vi "Chad Magic Voodoo 2.vi"() -> ()   [LabVIEW 2016]
panel:
  in  "Automatic Wire\n Feed not to Exceed":dbl=1.4
  in  "Add Wire Feed... (%)":dbl=4.0
  in  "For Every... (mm)":dbl=0.2
  out "W trigger Y":dbl
  out "C trigger Y":dbl
  out "R trigger Y":dbl
  in  "Window Bead Trigger heights":dbl[](array[numeric])
  in  "Robot Bead Trigger heights":dbl[](array[numeric])
  in  "Center Bead Trigger heights":dbl[](array[numeric])
  out "Shutter Open":bool
  in  "base path":path=path "C:/Users/Mark/Desktop/BeadScan"
  in  "Write Code":bool
  out "Bead3 Size":i32
  out "Bead2 Size":i32
  out "Bead1 Size":i32
  in  "Tab Control":T1(tab)
  in  "Mark Target Bead Height":bool
  out "All Beads":cluster{dbl[], dbl[]}[](graph)
  out "Target Bead Height":dbl
  in  "Set Correction C":bool
  in  "Set Trigger Offset":dbl
  in  "Center Bead Corrections":dbl[](array[numeric])
  in  "Center Bead Trigger Positions":dbl[](array[numeric])
  out "Center Bead #1":cluster{dbl[], dbl[]}[](graph)
  out "Center Bead Trigger":dbl
  in  "Set Trigger Center":bool
  in  "Undo":bool
  out "Difference From Bead Height Setpoint C":dbl
  out "Recommended % Change\n in Wire Feed C":dbl
  in  "Set Correction R":bool
  in  "Set Trigger Offset 2":dbl
  out "Robot Bead #2":cluster{dbl[], dbl[]}[](graph)
  in  "Robot Bead Trigger Positions":dbl[](array[numeric])
  in  "Robot Bead Corrections":dbl[](array[numeric])
  out "Robot Bead Trigger":dbl
  in  "Set Trigger Robot":bool
  in  "Undo":bool
  out "Difference From Bead Height Setpoint R":dbl
  out "Recommended % Change\n in Wire Feed R":dbl
  in  "Set Correction W":bool
  in  "Set Trigger Offset 3":dbl
  out "Window Bead #3":cluster{dbl[], dbl[]}[](graph)
  in  "Window Bead Trigger Positions":dbl[](array[numeric])
  in  "Window Bead Corrections":dbl[](array[numeric])
  out "Window Bead Trigger":dbl
  in  "Set Trigger Window":bool
  in  "Undo":bool
  out "Difference From Bead Height Setpoint W":dbl
  out "Recommended % Change\n in Wire Feed W":dbl
  in  "stop":bool
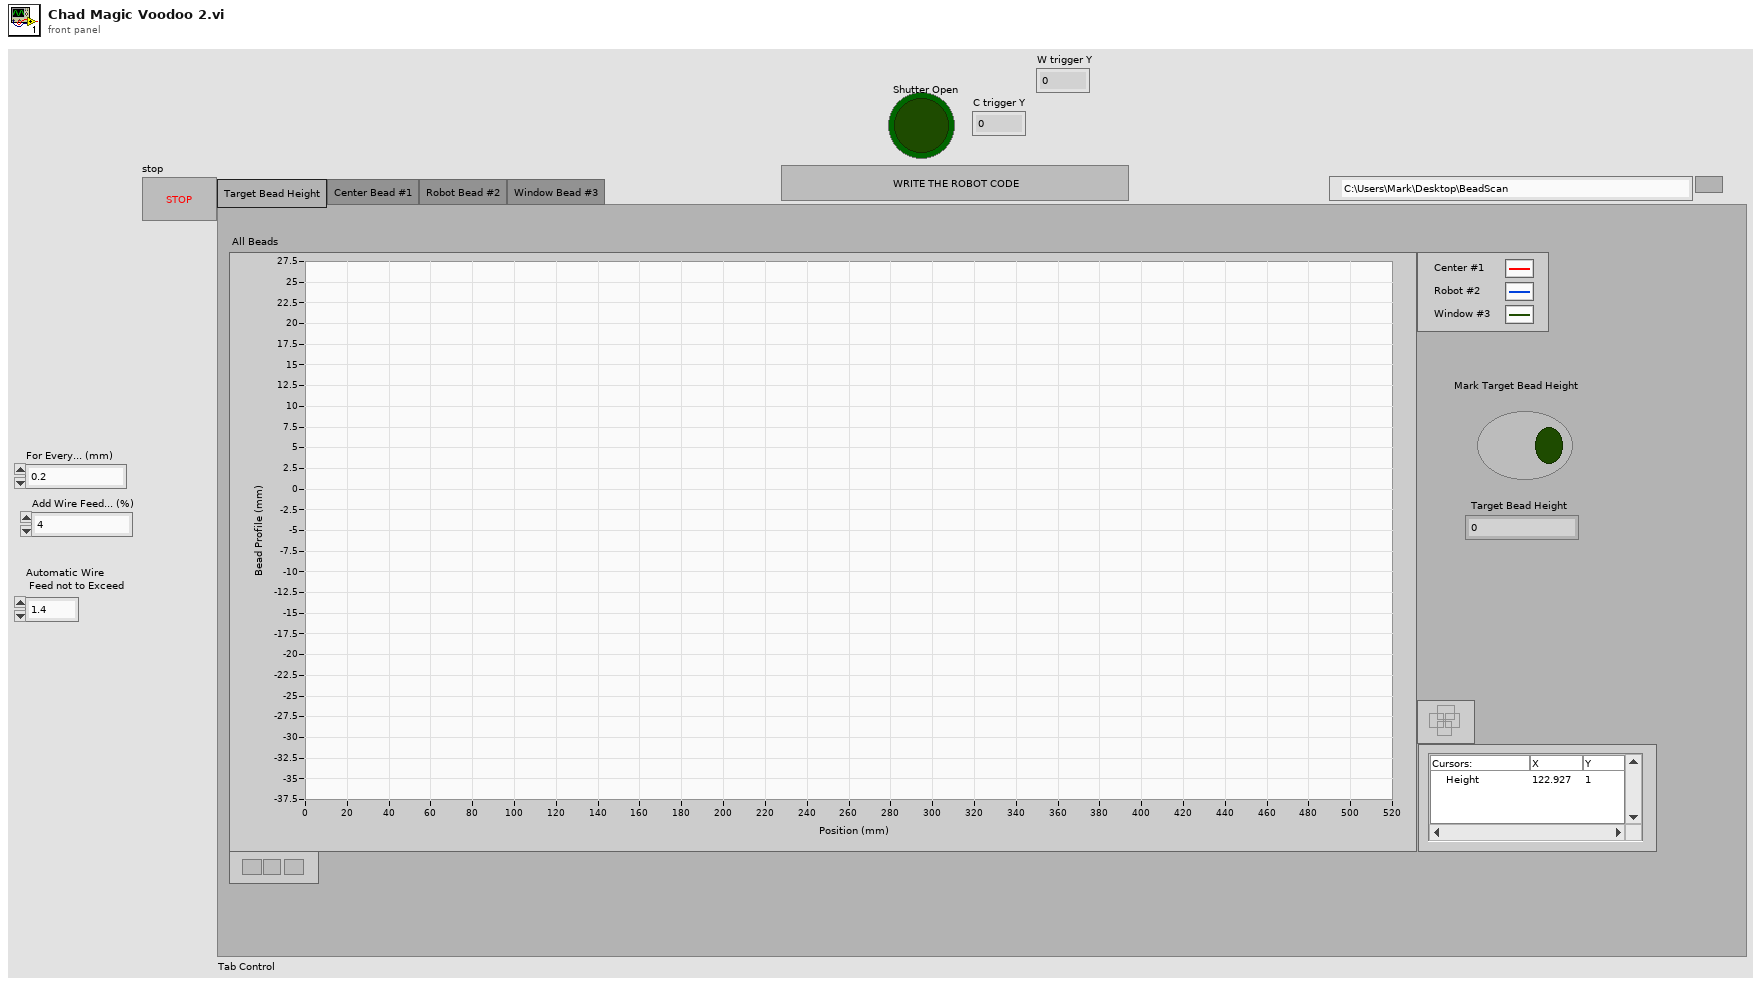
[diagram p1: front panel]
types:
  T1 = enum32{"Target Bead Height", "Center Bead #1", "Robot Bead #2", "Window Bead #3"}
  T2 = enum16{"open", "replace", "create", "open or create", "replace or create", "replace or create with confirmation"}
  T3 = cluster{"[0]":cluster{dbl[], dbl[]}, "[1]":cluster{dbl[], dbl[]}, "[2]":cluster{dbl[], dbl[]}}
  T4 = cluster{dbl[], "Center Bead Trigger heights":dbl[]}
  T5 = cluster{dbl[], "Window Bead Trigger heights":dbl[]}
  T6 = cluster{dbl[], "Robot Bead Trigger heights":dbl[]}
  T7 = cluster{dbl[], "Center Bead Trigger heights":dbl[]}[]
  T8 = cluster{dbl[], "Robot Bead Trigger heights":dbl[]}[]
  T9 = cluster{dbl[], "Window Bead Trigger heights":dbl[]}[]
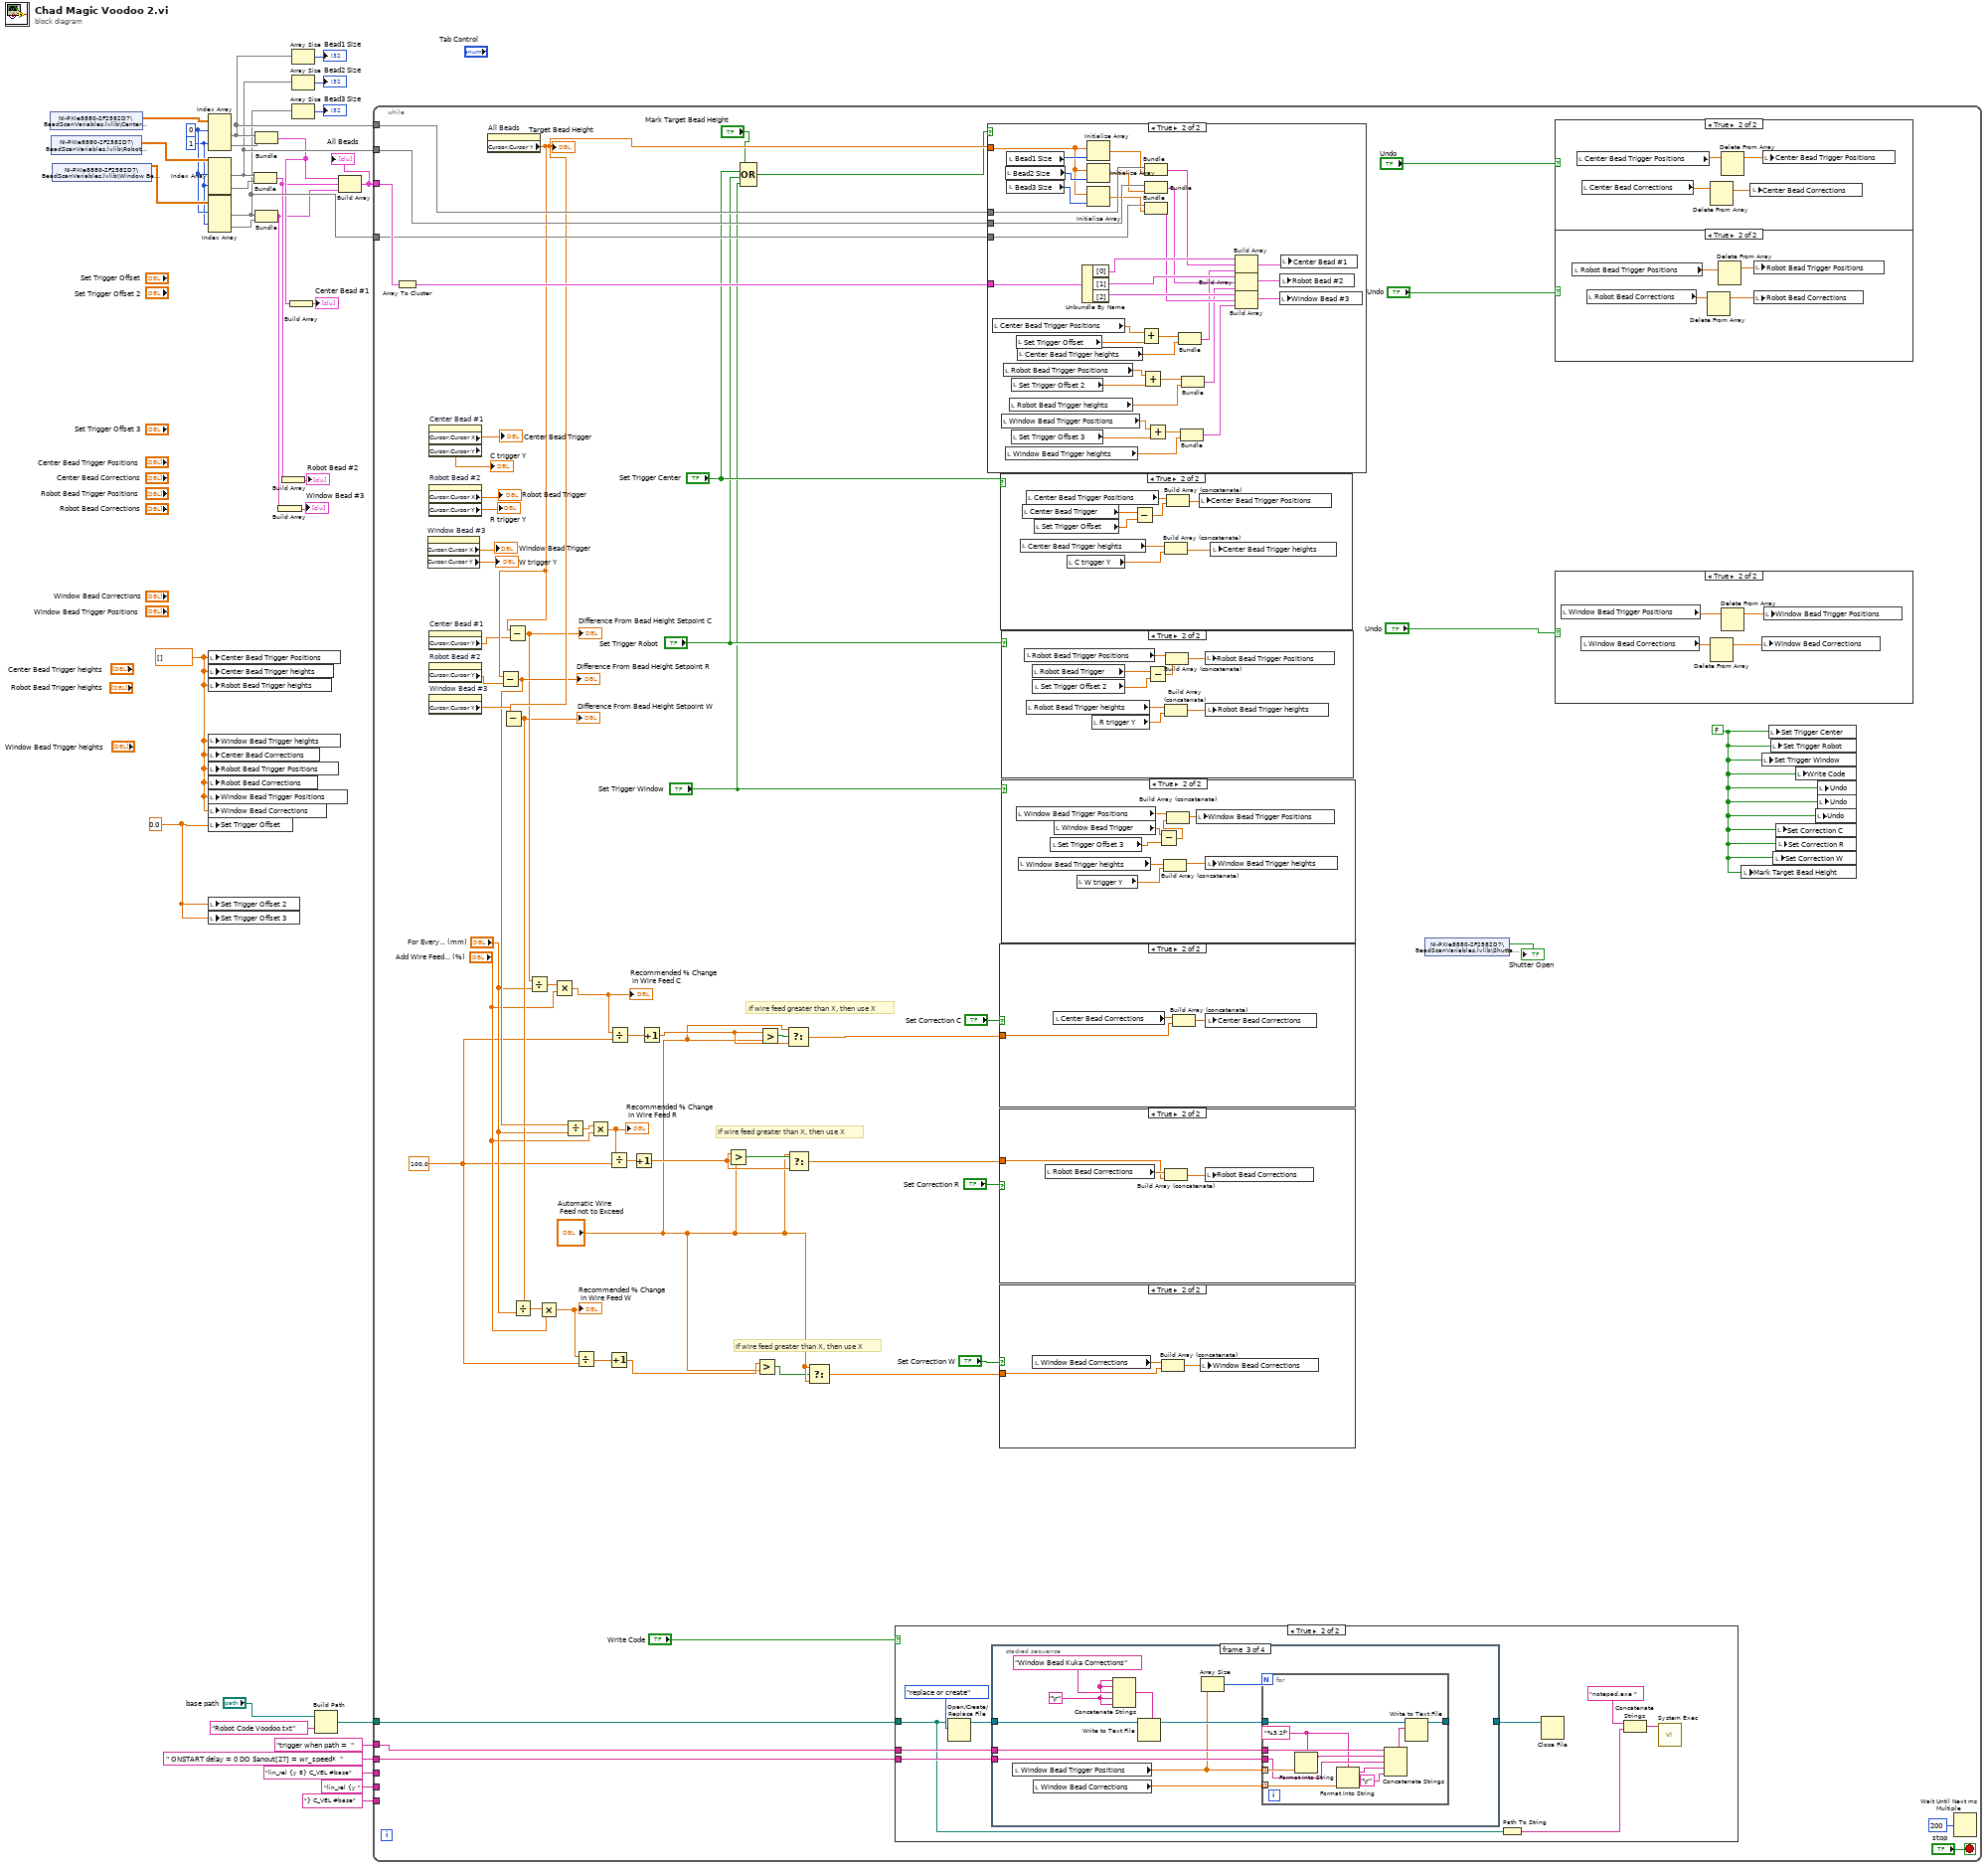
[diagram p0: block diagram]
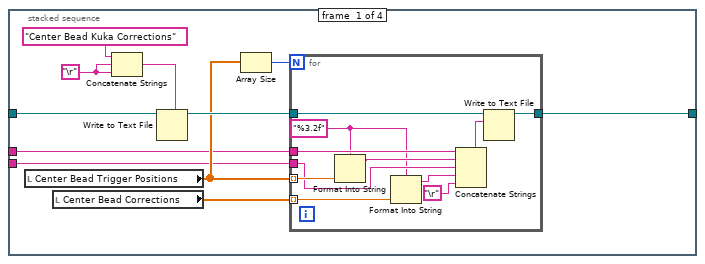
[diagram p6: hidden frame]
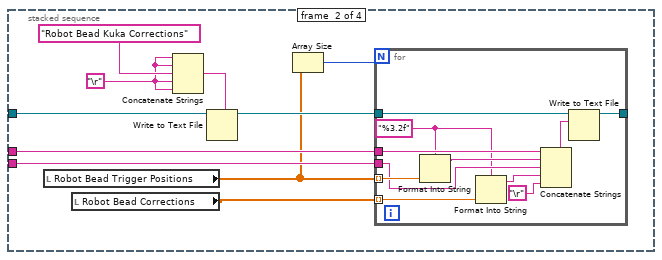
[diagram p7: hidden frame]
diagram:
  w2 = 0.0
  w1 = dbl[] []
  w26 = 1 ("index (row)")
  w27 = 0 ("index (row)")
  n1 = shared-variable "NI-PXIe8880-2F2582D7\\BeadScanVariables.lvlib\\Center Bead #1"() -> (w31:dbl[][])  [unwired: 1 in, 1 out]
  n2 = shared-variable "NI-PXIe8880-2F2582D7\\BeadScanVariables.lvlib\\Robot Bead #2"() -> (w29:dbl[][])  [unwired: 1 in, 1 out]
  n3 = shared-variable "NI-PXIe8880-2F2582D7\\BeadScanVariables.lvlib\\Window Bead #3"() -> (w28:dbl[][])  [unwired: 1 in, 1 out]
  n4 = Index Array(array=w31, index (row) #1=w27, index (row) #2=w26) -> (element #1=w19:dbl[], element #2=w30:dbl[])  [unwired: 2 in]
  n5 = Index Array(array=w29, index (row) #1=w27, index (row) #2=w26) -> (element #1=w18:dbl[], element #2=w25:dbl[])  [unwired: 2 in]
  n6 = Index Array(array=w28, index (row) #1=w27, index (row) #2=w26) -> (element #1=w17:dbl[], element #2=w24:dbl[])  [unwired: 2 in]
  n7 = local write "Center Bead Trigger Positions"(w1) -> ()
  n8 = local write "Center Bead Trigger heights"(w1) -> ()
  n9 = local write "Robot Bead Trigger heights"(w1) -> ()
  n10 = local write "Window Bead Trigger heights"(w1) -> ()
  n11 = local write "Center Bead Corrections"(w1) -> ()
  n12 = local write "Robot Bead Trigger Positions"(w1) -> ()
  n13 = local write "Robot Bead Corrections"(w1) -> ()
  n14 = local write "Window Bead Trigger Positions"(w1) -> ()
  n15 = local write "Window Bead Corrections"(w1) -> ()
  n16 = local write "Set Trigger Offset"(w2) -> ()
  n17 = local write "Set Trigger Offset 2"(w2) -> ()
  n18 = local write "Set Trigger Offset 3"(w2) -> ()
  n19 = Bundle(w18, w25) -> (w14:cluster{dbl[], dbl[]})  [unwired: 1 in]
  n20 = Bundle(w19, w30) -> (w15:cluster{dbl[], dbl[]})  [unwired: 1 in]
  n21 = Bundle(w17, w24) -> (w11:cluster{dbl[], dbl[]})  [unwired: 1 in]
  n22 = Build Array(w11) -> (→"Window Bead #3":cluster{dbl[], dbl[]}[])
  n23 = Build Array(w14) -> (→"Robot Bead #2":cluster{dbl[], dbl[]}[])
  n24 = Build Array(w15) -> (→"Center Bead #1":cluster{dbl[], dbl[]}[])
  n25 = Array Size(array=w19) -> (size(s)=→"Bead1 Size":i32)
  n26 = Array Size(array=w18) -> (size(s)=→"Bead2 Size":i32)
  n27 = Array Size(array=w17) -> (size(s)=→"Bead3 Size":i32)
  n28 = Build Path(base path="base path", name or relative path="Robot Code Voodoo.txt") -> (appended path=w8:path)
  n29 = Build Array(w15, w14, w11) -> (w20:cluster{dbl[], dbl[]}[])
  "All Beads" <- w20
  n30 = while {
    tunnel: w20 -> [w87]
    tunnel: w19 -> [w85]
    tunnel: w18 -> [w84]
    tunnel: w17 -> [w83]
    tunnel: w8 -> [w78]
    tunnel: "trigger when path =  " -> [w77]
    tunnel: " ONSTART delay = 0 DO $anout[27] = wr_speed*  " -> [w76]
    tunnel: "lin_rel {y 8} C_VEL #base" -> [_]
    tunnel: "lin_rel {y " -> [_]
    tunnel: "} C_VEL #base" -> [_]
    stop <- "stop" stop-if-true
    w46 = 100.0 ("y")
    w42 = FALSE
    # "If wire feed greater than X, then use X"
    # "If wire feed greater than X, then use X"
    # "If wire feed greater than X, then use X"
    n31 = Array To Cluster(array=w87) -> (cluster=w86:T3)
    n32 = property on="Window Bead #3" class="XYGraph (strict)"() -> ("Cursor.Cursor X"=→"Window Bead Trigger":dbl, "Cursor.Cursor Y"=→"W trigger Y":dbl)  [unwired: 2 in, 2 out]
    n33 = property on="Center Bead #1" class="XYGraph (strict)"() -> ("Cursor.Cursor X"=→"Center Bead Trigger":dbl, "Cursor.Cursor Y"=→"C trigger Y":dbl)  [unwired: 2 in, 2 out]
    n34 = property on="Robot Bead #2" class="XYGraph (strict)"() -> ("Cursor.Cursor X"=→"Robot Bead Trigger":dbl, "Cursor.Cursor Y"=→"R trigger Y":dbl)  [unwired: 2 in, 2 out]
    n35 = property on="Center Bead #1" class="XYGraph (strict)"() -> ("Cursor.Cursor Y"=w72:dbl)  [unwired: 2 in, 2 out]
    n36 = property on="Robot Bead #2" class="XYGraph (strict)"() -> ("Cursor.Cursor Y"=w71:dbl)  [unwired: 2 in, 2 out]
    n37 = property on="Window Bead #3" class="XYGraph (strict)"() -> ("Cursor.Cursor Y"=w70:dbl)  [unwired: 2 in, 2 out]
    n38 = property on="All Beads" class="XYGraph (strict)"() -> ("Cursor.Cursor Y"=w73:dbl)  [unwired: 2 in, 2 out]
    "Target Bead Height" <- w73
    n39 = Subtract(x=w73, y=w71) -> (x-y=w58:dbl)
    "Difference From Bead Height Setpoint R" <- w58
    n40 = Subtract(x=w73, y=w70) -> (x-y=w55:dbl)
    "Difference From Bead Height Setpoint W" <- w55
    n41 = Subtract(x=w73, y=w72) -> (x-y=w56:dbl)
    "Difference From Bead Height Setpoint C" <- w56
    n42 = Divide(x=w55, y="For Every... (mm)") -> (x/y=w59:dbl)
    n43 = Divide(x=w56, y="For Every... (mm)") -> (x/y=w57:dbl)
    n44 = Multiply(x=w59, y="Add Wire Feed... (%)") -> (x*y=w47:dbl)
    "Recommended % Change\n in Wire Feed W" <- w47
    n45 = Multiply(x=w57, y="Add Wire Feed... (%)") -> (x*y=w48:dbl)
    "Recommended % Change\n in Wire Feed C" <- w48
    n46 = Divide(x=w58, y="For Every... (mm)") -> (x/y=w60:dbl)
    n47 = Divide(x=w47, y=w46) -> (x/y=w43:dbl)
    n48 = Multiply(x=w60, y="Add Wire Feed... (%)") -> (x*y=w49:dbl)
    "Recommended % Change\n in Wire Feed R" <- w49
    n49 = Divide(x=w49, y=w46) -> (x/y=w45:dbl)
    n50 = Increment(x=w43) -> (x+1=w41:dbl)
    n51 = Divide(x=w48, y=w46) -> (x/y=w44:dbl)
    n52 = Increment(x=w45) -> (x+1=w36:dbl)
    n53 = Increment(x=w44) -> (x+1=w40:dbl)
    n54 = Greater?(x=w36, y="Automatic Wire\n Feed not to Exceed") -> (0:w37:bool)
    n55 = Compound Arithmetic op=OR("Mark Target Bead Height", "Set Trigger Center", "Set Trigger Robot", "Set Trigger Window") -> (w64:bool)
    n56 = Greater?(x=w41, y="Automatic Wire\n Feed not to Exceed") -> (0:w33:bool)
    n57 = Greater?(x=w40, y="Automatic Wire\n Feed not to Exceed") -> (0:w39:bool)
    n58 = Select(t="Automatic Wire\n Feed not to Exceed", s=w39, f=w40) -> (s? t:f=w38:dbl)
    n59 = Select(t="Automatic Wire\n Feed not to Exceed", s=w37, f=w36) -> (s? t:f=w35:dbl)
    n60 = Select(t="Automatic Wire\n Feed not to Exceed", s=w33, f="Automatic Wire\n Feed not to Exceed") -> (s? t:f=w32:dbl)
    n61 = case shown="True" "Write Code" {
      tunnel: w78 -> [_ w100]
      tunnel: w77 -> [_ w107]
      tunnel: w76 -> [_ w106]
      frame False {
      }
      frame True {
        n62 = Open/Create/Replace File(file path (use dialog)=w100, operation (0:open)=T2."replace or create") -> (refnum out=w108:refnum<file>)  [unwired: 4 in, 2 out]
        n63 = stacked-sequence {
          tunnel: w108 -> [w116 w137 w158 _]
          tunnel: w107 -> [w111 w135 w156 _]
          tunnel: w106 -> [w110 w134 w155 _]
          tunnel: [w109 _ _ _] -> w105
          frame #0 {
            w118 = "\r"
            n64 = local read "Center Bead Trigger Positions"() -> (w113:dbl[])
            n65 = local read "Center Bead Corrections"() -> (w112:dbl[])
            n66 = Concatenate Strings("Center Bead Kuka Corrections", w118, w118) -> (w117:string)
            n67 = Write to Text File(file (use dialog)=w116, text=w117) -> (refnum out=w115:refnum<file>)  [unwired: 2 in, 2 out]
            n68 = Array Size(array=w113) -> (size(s)=w114:i32)
            n69 = for {
              N: w114 -> [_]
              tunnel: w115 -> [w130]
              tunnel: w113 -> [w127] mode=indexing
              tunnel: w112 -> [w124] mode=indexing
              tunnel: w111 -> [w129]
              tunnel: w110 -> [w125]
              tunnel: [w122] -> w109
              w121 = "%3.2f" ("format string")
              n70 = Format Into String(format string=w121, w127) -> (resulting string=w128:string)  [unwired: 2 in, 1 out]
              n71 = Format Into String(format string=w121, w124) -> (resulting string=w123:string)  [unwired: 2 in, 1 out]
              n72 = Concatenate Strings(w129, w128, w125, w123, "\r") -> (w126:string)
              n73 = Write to Text File(file (use dialog)=w130, text=w126) -> (refnum out=w122:refnum<file>)  [unwired: 2 in, 2 out]
            }
          }
          frame #1 {
            w131 = "\r"
            n74 = local read "Robot Bead Trigger Positions"() -> (w132:dbl[])
            n75 = local read "Robot Bead Corrections"() -> (w133:dbl[])
            n76 = Concatenate Strings(w131, w131, "Robot Bead Kuka Corrections", w131, w131) -> (w139:string)
            n77 = Write to Text File(file (use dialog)=w137, text=w139) -> (refnum out=w138:refnum<file>)  [unwired: 2 in, 2 out]
            n78 = Array Size(array=w132) -> (size(s)=w136:i32)
            n79 = for {
              N: w136 -> [_]
              tunnel: w138 -> [w151]
              tunnel: w132 -> [w148] mode=indexing
              tunnel: w133 -> [w145] mode=indexing
              tunnel: w135 -> [w150]
              tunnel: w134 -> [w146]
              tunnel: [w143] -> _
              w142 = "%3.2f" ("format string")
              n80 = Format Into String(format string=w142, w148) -> (resulting string=w149:string)  [unwired: 2 in, 1 out]
              n81 = Format Into String(format string=w142, w145) -> (resulting string=w144:string)  [unwired: 2 in, 1 out]
              n82 = Concatenate Strings(w150, w149, w146, w144, "\r") -> (w147:string)
              n83 = Write to Text File(file (use dialog)=w151, text=w147) -> (refnum out=w143:refnum<file>)  [unwired: 2 in, 2 out]
            }
          }
          frame #2 {
            w152 = "\r"
            n84 = local read "Window Bead Trigger Positions"() -> (w153:dbl[])
            n85 = local read "Window Bead Corrections"() -> (w154:dbl[])
            n86 = Concatenate Strings(w152, w152, "Window Bead Kuka Corrections", w152, w152) -> (w160:string)
            n87 = Write to Text File(file (use dialog)=w158, text=w160) -> (refnum out=w159:refnum<file>)  [unwired: 2 in, 2 out]
            n88 = Array Size(array=w153) -> (size(s)=w157:i32)
            n89 = for {
              N: w157 -> [_]
              tunnel: w159 -> [w172]
              tunnel: w153 -> [w169] mode=indexing
              tunnel: w154 -> [w166] mode=indexing
              tunnel: w156 -> [w171]
              tunnel: w155 -> [w167]
              tunnel: [w164] -> _
              w163 = "%3.2f" ("format string")
              n90 = Format Into String(format string=w163, w169) -> (resulting string=w170:string)  [unwired: 2 in, 1 out]
              n91 = Format Into String(format string=w163, w166) -> (resulting string=w165:string)  [unwired: 2 in, 1 out]
              n92 = Concatenate Strings(w171, w170, w167, w165, "\r") -> (w168:string)
              n93 = Write to Text File(file (use dialog)=w172, text=w168) -> (refnum out=w164:refnum<file>)  [unwired: 2 in, 2 out]
            }
          }
          frame #3 {
          }
        }
        n94 = Path To String(path=w100) -> (string=w101:string)
        n95 = Close File(refnum=w105) -> ()  [unwired: 1 in, 2 out]
        n96 = Concatenate Strings("notepad.exe " ("command line"), w101) -> (w103:string)
        n97 = call <vilib>:"System Exec.vi"("command line"=w103) -> ()  [unwired: 7 in, 4 out]
      }
    }
    n98 = case shown="True" w64 {
      tunnel: w73 -> [_ w241]
      tunnel: w86 -> [_ w239]
      tunnel: w85 -> [_ w238]
      tunnel: w84 -> [_ w236]
      tunnel: w83 -> [_ w235]
      frame False {
      }
      frame True {
        n99 = local read "Center Bead Trigger Positions"() -> (w219:dbl[])
        n100 = local read "Window Bead Trigger Positions"() -> (w213:dbl[])
        n101 = local read "Robot Bead Trigger Positions"() -> (w216:dbl[])
        n102 = local read "Bead2 Size"() -> (w242:i32)
        n103 = local read "Window Bead Trigger heights"() -> (w212:dbl[])
        n104 = local read "Bead1 Size"() -> (w243:i32)
        n105 = local read "Bead3 Size"() -> (w240:i32)
        n106 = local read "Robot Bead Trigger heights"() -> (w214:dbl[])
        n107 = local read "Set Trigger Offset 2"() -> (w222:dbl)
        n108 = local read "Set Trigger Offset 3"() -> (w221:dbl)
        n109 = local read "Set Trigger Offset"() -> (w223:dbl)
        n110 = local read "Center Bead Trigger heights"() -> (w217:dbl[])
        n111 = Unbundle By Name(w239) -> ("[0]"=w232:cluster{dbl[], dbl[]}, "[1]"=w230:cluster{dbl[], dbl[]}, "[2]"=w228:cluster{dbl[], dbl[]})
        n112 = Initialize Array(w241, w243) -> (w237:dbl[])
        n113 = Initialize Array(w241, w242) -> (w233:dbl[])
        n114 = Initialize Array(w241, w240) -> (w234:dbl[])
        n115 = Add(x=w219, y=w223) -> (x+y=w218:dbl[])
        n116 = Add(x=w216, y=w222) -> (x+y=w215:dbl[])
        n117 = Bundle(w238, w237) -> (w231:cluster{dbl[], dbl[]})  [unwired: 1 in]
        n118 = Bundle(w236, w233) -> (w229:cluster{dbl[], dbl[]})  [unwired: 1 in]
        n119 = Bundle(w235, w234) -> (w227:cluster{dbl[], dbl[]})  [unwired: 1 in]
        n120 = Add(x=w213, y=w221) -> (x+y=w220:dbl[])
        n121 = Bundle(w218, "Center Bead Trigger heights"=w217) -> (w211:T4)  [unwired: 1 in]
        n122 = Bundle(w220, "Window Bead Trigger heights"=w212) -> (w209:T5)  [unwired: 1 in]
        n123 = Bundle(w215, "Robot Bead Trigger heights"=w214) -> (w210:T6)  [unwired: 1 in]
        n124 = Build Array(w232, w231, w211) -> (w226:T7)
        n125 = Build Array(w230, w229, w210) -> (w225:T8)
        n126 = Build Array(w228, w227, w209) -> (w224:T9)
        n127 = local write "Window Bead #3"(w224) -> ()
        n128 = local write "Robot Bead #2"(w225) -> ()
        n129 = local write "Center Bead #1"(w226) -> ()
      }
    }
    n130 = case shown="True" "Set Correction C" {
      tunnel: w38 -> [_ w97]
      frame False {
      }
      frame True {
        n131 = local read "Center Bead Corrections"() -> (w99:dbl[])
        n132 = Build Array (concatenate)(w99, w97) -> (w98:dbl[])
        n133 = local write "Center Bead Corrections"(w98) -> ()
      }
    }
    n134 = case shown="True" "Set Correction R" {
      tunnel: w35 -> [_ w94]
      frame False {
      }
      frame True {
        n135 = local read "Robot Bead Corrections"() -> (w96:dbl[])
        n136 = Build Array (concatenate)(w96, w94) -> (w95:dbl[])
        n137 = local write "Robot Bead Corrections"(w95) -> ()
      }
    }
    n138 = case shown="True" "Set Correction W" {
      tunnel: w32 -> [_ w91]
      frame False {
      }
      frame True {
        n139 = local read "Window Bead Corrections"() -> (w93:dbl[])
        n140 = Build Array (concatenate)(w93, w91) -> (w92:dbl[])
        n141 = local write "Window Bead Corrections"(w92) -> ()
      }
    }
    n142 = case shown="True" "Set Trigger Center" {
      frame False {
      }
      frame True {
        n143 = local read "Center Bead Trigger heights"() -> (w203:dbl[])
        n144 = local read "Center Bead Trigger"() -> (w206:dbl)
        n145 = local read "Center Bead Trigger Positions"() -> (w208:dbl[])
        n146 = local read "Set Trigger Offset"() -> (w204:dbl)
        n147 = local read "C trigger Y"() -> (w202:dbl)
        n148 = Subtract(x=w206, y=w204) -> (x-y=w205:dbl)
        n149 = Build Array (concatenate)(w203, w202) -> (w201:dbl[])
        n150 = Build Array (concatenate)(w208, w205) -> (w207:dbl[])
        n151 = local write "Center Bead Trigger Positions"(w207) -> ()
        n152 = local write "Center Bead Trigger heights"(w201) -> ()
      }
    }
    n153 = case shown="True" "Set Trigger Robot" {
      frame False {
      }
      frame True {
        n154 = local read "Robot Bead Trigger Positions"() -> (w200:dbl[])
        n155 = local read "Robot Bead Trigger heights"() -> (w194:dbl[])
        n156 = local read "Robot Bead Trigger"() -> (w198:dbl)
        n157 = local read "Set Trigger Offset 2"() -> (w196:dbl)
        n158 = local read "R trigger Y"() -> (w193:dbl)
        n159 = Subtract(x=w198, y=w196) -> (x-y=w197:dbl)
        n160 = Build Array (concatenate)(w194, w193) -> (w195:dbl[])
        n161 = Build Array (concatenate)(w200, w197) -> (w199:dbl[])
        n162 = local write "Robot Bead Trigger Positions"(w199) -> ()
        n163 = local write "Robot Bead Trigger heights"(w195) -> ()
      }
    }
    n164 = case shown="True" "Set Trigger Window" {
      frame False {
      }
      frame True {
        n165 = local read "Window Bead Trigger Positions"() -> (w192:dbl[])
        n166 = local read "Window Bead Trigger heights"() -> (w187:dbl[])
        n167 = local read "Set Trigger Offset 3"() -> (w190:dbl)
        n168 = local read "Window Bead Trigger"() -> (w189:dbl)
        n169 = local read "W trigger Y"() -> (w186:dbl)
        n170 = Subtract(x=w189, y=w190) -> (x-y=w188:dbl)
        n171 = Build Array (concatenate)(w187, w186) -> (w185:dbl[])
        n172 = Build Array (concatenate)(w192, w188) -> (w191:dbl[])
        n173 = local write "Window Bead Trigger Positions"(w191) -> ()
        n174 = local write "Window Bead Trigger heights"(w185) -> ()
      }
    }
    n175 = shared-variable "NI-PXIe8880-2F2582D7\\BeadScanVariables.lvlib\\Shutter Open"() -> (→"Shutter Open":bool)  [unwired: 1 in, 1 out]
    n176 = case shown="True" "Undo" {
      frame False {
      }
      frame True {
        n177 = local read "Robot Bead Trigger Positions"() -> (w179:dbl[])
        n178 = local read "Robot Bead Corrections"() -> (w180:dbl[])
        n179 = Delete From Array(array=w180) -> (array with subset deleted=w177:dbl[])  [unwired: 2 in, 1 out]
        n180 = Delete From Array(array=w179) -> (array with subset deleted=w178:dbl[])  [unwired: 2 in, 1 out]
        n181 = local write "Robot Bead Trigger Positions"(w178) -> ()
        n182 = local write "Robot Bead Corrections"(w177) -> ()
      }
    }
    n183 = case shown="True" "Undo" {
      frame False {
      }
      frame True {
        n184 = local read "Window Bead Trigger Positions"() -> (w175:dbl[])
        n185 = local read "Window Bead Corrections"() -> (w174:dbl[])
        n186 = Delete From Array(array=w174) -> (array with subset deleted=w173:dbl[])  [unwired: 2 in, 1 out]
        n187 = Delete From Array(array=w175) -> (array with subset deleted=w176:dbl[])  [unwired: 2 in, 1 out]
        n188 = local write "Window Bead Corrections"(w173) -> ()
        n189 = local write "Window Bead Trigger Positions"(w176) -> ()
      }
    }
    n190 = case shown="True" "Undo" {
      frame False {
      }
      frame True {
        n191 = local read "Center Bead Trigger Positions"() -> (w183:dbl[])
        n192 = local read "Center Bead Corrections"() -> (w182:dbl[])
        n193 = Delete From Array(array=w182) -> (array with subset deleted=w181:dbl[])  [unwired: 2 in, 1 out]
        n194 = Delete From Array(array=w183) -> (array with subset deleted=w184:dbl[])  [unwired: 2 in, 1 out]
        n195 = local write "Center Bead Corrections"(w181) -> ()
        n196 = local write "Center Bead Trigger Positions"(w184) -> ()
      }
    }
    n197 = local write "Mark Target Bead Height"(w42) -> ()
    n198 = local write "Set Trigger Window"(w42) -> ()
    n199 = local write "Set Trigger Center"(w42) -> ()
    n200 = local write "Set Trigger Robot"(w42) -> ()
    n201 = local write "Set Correction W"(w42) -> ()
    n202 = local write "Set Correction C"(w42) -> ()
    n203 = local write "Set Correction R"(w42) -> ()
    n204 = local write "Write Code"(w42) -> ()
    n205 = local write "Undo"(w42) -> ()
    n206 = local write "Undo"(w42) -> ()
    n207 = local write "Undo"(w42) -> ()
    n208 = Wait Until Next ms Multiple(millisecond multiple=u32 200) -> ()  [unwired: 1 out]
  }
